vi "Load Analog Replay.vi"(6 "memory":refnum<k21>="Replay Memory 0", 11 "load input.<user name>":T1={"Data"=[0, 0, 0, 0, 0, 0, 0, 0, 0, 0, 0, 0, 0, 0, 0, 0], "LoadOffset"=0, "Done"=FALSE}) -> (0 "done":bool)   [LabVIEW 2015, in "Engine Simulation Toolkit.lvlib" / "Analog Replay.lvlib"]
doc: "Loads data from NI VeriStand into the analog replay memory. <b> This VI should be in an SCTL</b>\n\n<b>load input.<user name></b> - input for the component. NI VeriStand will set these values. create a control for this input. Replace <user name> with the name you wish this component to display as inside NI VeriStand. Make this name consistent for all controls, indicators, for all VIs of this component.\n<b>memory</b> - reference to an I16 memory of size 2^N where N must be a value 10 to 16. Recommended size is 14. The memory can be set to never arbitrate to save resources. This reference should also be wired to Analog Replay.vi\n\n<b>done</b> - done loading signal. Wire this to the SCTL stop terminal."
uses:
  Analog Replay.lvlib
  Load Input.ctl
  <vilib>/rvi/Emulation/niFpgaSctlEmulationGetInTimedLoop.vi
  <vilib>/Utility/error.llb/Clear Errors.vi
  <vilib>/rvi/DataTransferAndStorage/Container/Common/niFpgaContainerExecOnDevCompGetState.vi
  <vilib>/rvi/Emulation/niFpgaEmulationIsFPGAContextNoSignature.vi
  <vilib>/rvi/DataTransferAndStorage/Container/Common/niFpgaContainerGetUniqueNameForEmu.vi
  <vilib>/rvi/Emulation/niFpgaProcessEmulError.vi
  <vilib>/rvi/errors/nirviReportUnexpectedCaseInternalError (U32).vi
  <vilib>/rvi/Memory/Memory_Emulation/niFpgaMemoryEmulationCacheClearOnFirstRun.vi
  <vilib>/rvi/Memory/Memory_Emulation/nirvimemoryEmulationManagerCache_MakeExclusive.vi
  <vilib>/rvi/Memory/Memory_Emulation/niFpgaMemoryEmulationValidateCache.vi
  <vilib>/rvi/Memory/Memory_Emulation/nirvimemoryEmulationManagerCache_InsertValue.vi
  <vilib>/rvi/Memory/Memory_Emulation/nirvimemoryEmulationManagerCache_ReleaseExclusive.vi
  <vilib>/rvi/Memory/Memory_Emulation/nirvimemoryEmulationManagerCache_GetValue.vi
  <vilib>/rvi/Memory/Memory_Emulation/nirvimemoryEmulationManagerCache_SetValue.vi
  <vilib>/rvi/Emulation/niFpgaSctlEmulationResourceMgr.vi
  <vilib>/rvi/DataTransferAndStorage/Container/XNode/niFpgaContainer.xnode
  <vilib>/rvi/Memory/Memory_Emulation/niFpgaMemoryEmulationRefIn.vi
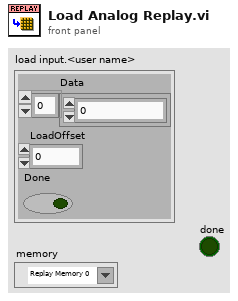
[diagram p1: front panel]
types:
  T1 = typedef "Engine Simulation Toolkit.lvlib/Analog Replay.lvlib/Load Input.ctl" = cluster{"Data":i16[], "LoadOffset":u16, "Done":bool}
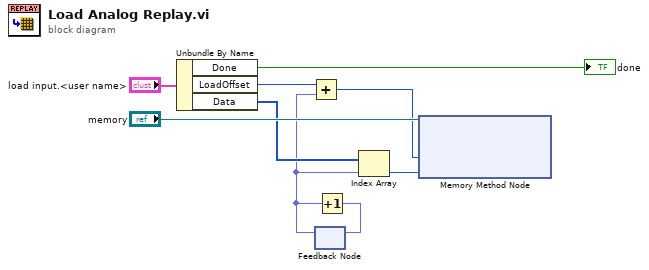
[diagram p0: block diagram]
diagram:
  n1 = Unbundle By Name("load input.<user name>") -> ("Done"=→"done":bool, "LoadOffset"=w5:u16, "Data"=w7:i16[])
  n2 = feedback #1() -> (w3:fxp<+,4,4>)  [unwired: 1 in]
  n3 = Add(x=w5, y=w3) -> (x+y=w2:u16)
  n4 = Increment(x=w3) -> (x+1=w1:fxp<+,4,4>)
  n5 = feedback-in #1(w1) -> ()
  n6 = Index Array(array=w7, index=w3) -> (element=w4:i16)
  n7 = xnode ("Memory Method Node")("Address"=w2, "Data"=w4, "Memory In"="memory") -> ()  [unwired: 1 out]
